vi "CRYConvertWorkinValue.vi"(6 "no ppk?":bool=TRUE, 8 "Work in":u16, 10 "In":T1={"Name"="", "Curve"=[], "X data"=1, "Y data"=1, "Z data"=1, "X axis"=0, "Y axis"=1, "Z axis"=1, "X unit"="Hz", "Y unit"="", "Z unit"="deg.", "X dB ref"=1.0, "Y dB ref"=1.0, "Z dB ref"=1.0, "single val"=FALSE, "protected"=FALSE, "display X"=TRUE, "display Y"=TRUE, "display Z"=TRUE, "Test Info"="", "Step No."=0, "Plot Settings"={"Color"=0, "Interpolation"=0, "Point Style"=0, "Line Style"=0, "Point Color"=0, "Line Width"=0, "Bar Plot Style"=0, "Fill To"=0}, "AutoProtect"=FALSE} {"Z data" items=["dB", "Lin"]; "X data" items=["dB", "Lin"]; "Y data" items=["dB", "Lin"]; "Z dB ref" format="%.1f"; "Z axis" items=["Log", "Lin"]; "X dB ref" format="%.1f"; "X axis" items=["Log", "Lin"]; "Y axis" items=["Log", "Lin"]; "Y dB ref" format="%.1f"; "Curve"."z" format="%.2f"; "Curve"."y" format="%.2f"; "Curve"."x" format="%.2f"}, 11 "Type":u16(slide) caption="Type:") -> (1 "Out":T1={"Name"="", "Curve"=[], "X data"=1, "Y data"=1, "Z data"=1, "X axis"=0, "Y axis"=1, "Z axis"=1, "X unit"="Hz", "Y unit"="", "Z unit"="deg.", "X dB ref"=1.0, "Y dB ref"=1.0, "Z dB ref"=1.0, "single val"=FALSE, "protected"=FALSE, "display X"=TRUE, "display Y"=TRUE, "display Z"=TRUE, "Test Info"="", "Step No."=0, "Plot Settings"={"Color"=0, "Interpolation"=0, "Point Style"=0, "Line Style"=0, "Point Color"=0, "Line Width"=0, "Bar Plot Style"=0, "Fill To"=0}, "AutoProtect"=FALSE} {"Z data" items=["dB", "Lin"]; "X data" items=["dB", "Lin"]; "Y data" items=["dB", "Lin"]; "Z dB ref" format="%.1f"; "Z axis" items=["Log", "Lin"]; "X dB ref" format="%.1f"; "X axis" items=["Log", "Lin"]; "Y axis" items=["Log", "Lin"]; "Y dB ref" format="%.1f"; "Curve"."z" format="%.2f"; "Curve"."y" format="%.2f"; "Curve"."x" format="%.2f"})   [LabVIEW 2013]
uses:
  Typedef Control/CRYData Cluster.ctl
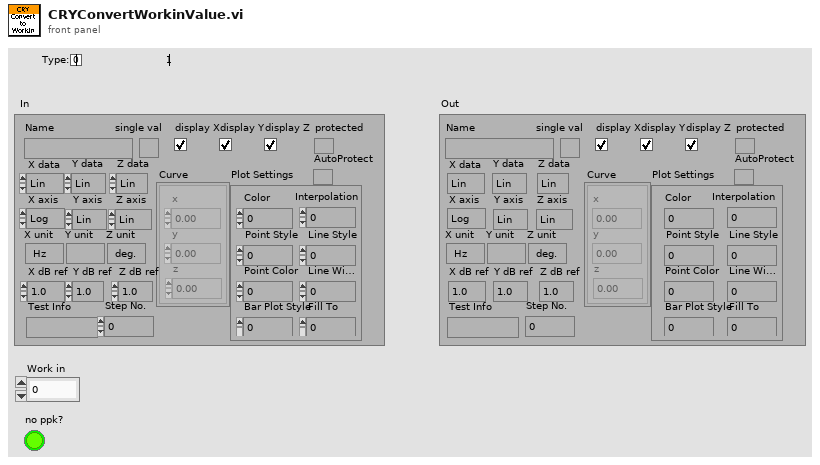
[diagram p1: front panel]
types:
  T1 = typedef "CRYData Cluster.ctl" = cluster{"Name":string, "Curve":cluster{"x":dbl, "y":dbl, "z":dbl}[], "X data":u16, "Y data":u16, "Z data":u16, "X axis":u16, "Y axis":u16, "Z axis":u16, "X unit":string, "Y unit":string, "Z unit":string, "X dB ref":dbl, "Y dB ref":dbl, "Z dB ref":dbl, "single val":bool, "protected":bool, "display X":bool, "display Y":bool, "display Z":bool, "Test Info":string, "Step No.":i32, "Plot Settings":cluster{"Color":u32, "Interpolation":u8, "Point Style":u8, "Line Style":u8, "Point Color":u32, "Line Width":u8, "Bar Plot Style":u8, "Fill To":i16}, "AutoProtect":bool}
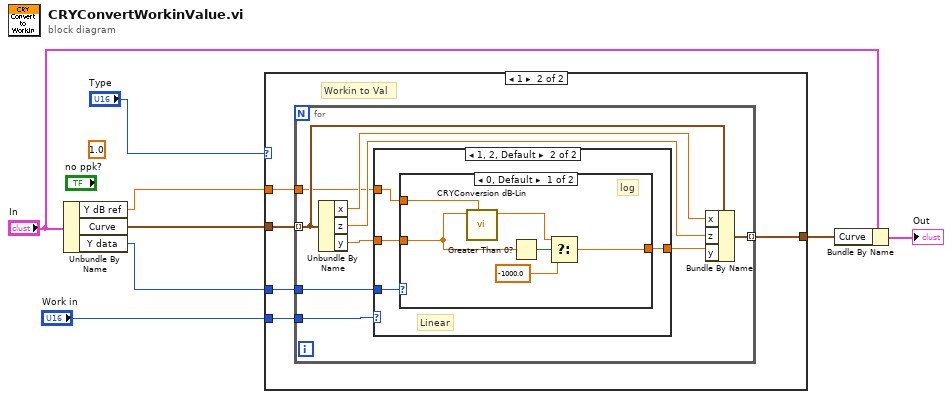
[diagram p0: block diagram]
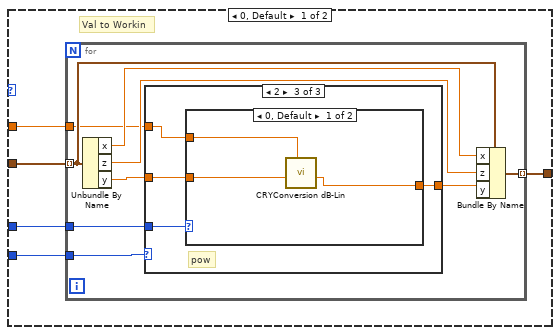
[diagram p2: hidden frame]
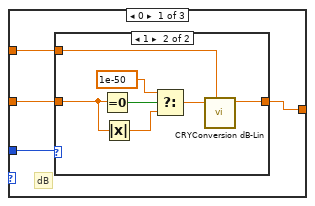
[diagram p3: hidden frame]
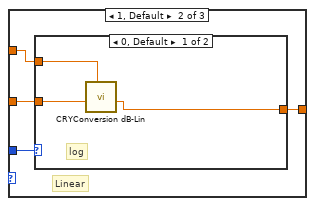
[diagram p5: hidden frame]
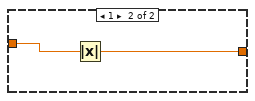
[diagram p7: hidden frame]
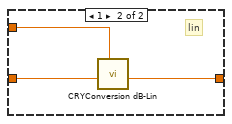
[diagram p9: hidden frame]
diagram:
  (unwired) 1.0 ("Y dB ref")
  n1 = Unbundle By Name("In") -> ("Y dB ref"=w1:dbl, "Curve"=w8:cluster{"x":dbl, "y":dbl, "z":dbl}[], "Y data"=w6:u16)
  n2 = case shown="1" "Type" {
    tunnel: w8 -> [w13 w56]
    tunnel: "Work in" -> [w10 w55]
    tunnel: w6 -> [w11 w54]
    tunnel: [w9 w53] -> w4
    tunnel: w1 -> [w12 w52]
    frame 0, Default {
      # "Val to Workin"
      n3 = for {
        tunnel: w13 -> [w18] mode=indexing
        tunnel: w10 -> [w22]
        tunnel: w11 -> [w20]
        tunnel: [w15] -> w9 mode=indexing
        tunnel: w12 -> [w14]
        n4 = Unbundle By Name(w18) -> ("x"=w19:dbl, "z"=w17:dbl, "y"=w21:dbl)
        n5 = case shown="2" w22 {
          tunnel: w21 -> [w26 w36 w43]
          tunnel: [w25 w37 w45] -> w16
          tunnel: w20 -> [w24 w38 w46]
          tunnel: w14 -> [w23 w35 w44]
          frame 0 {
            # "dB"
            n6 = case shown="1" w24 {
              tunnel: w26 -> [w27 w32]
              tunnel: [w27 w28] -> w25
              tunnel: w23 -> [_ w31]
              frame 0, Default {
              }
              frame 1 {
                n7 = Equal To 0?(x=w32) -> (x = 0?=w34:bool)
                n8 = Absolute Value(x=w32) -> (abs(x)=w30:dbl)
                n9 = Select(t=1e-50, s=w34, f=w30) -> (s? t:f=w29:dbl)
                n10 = call "CRYConversion dB-Lin.vi"("dB ref."=w31, "Lin In"=w29) -> ("Log Out"=w28:dbl)  [unwired: 4 in, 3 out]
              }
            }
          }
          frame 1, Default {
            # "Linear"
            n11 = case shown="0, Default" w38 {
              tunnel: [w39 w42] -> w37
              tunnel: w36 -> [w40 w42]
              tunnel: w35 -> [w41 _]
              frame 0, Default {
                # "log"
                n12 = call "CRYConversion dB-Lin.vi"("dB ref."=w41, "Log In"=w40) -> ("Lin Out"=w39:dbl)  [unwired: 4 in, 3 out]
              }
              frame 1 {
                # "lin"
              }
            }
          }
          frame 2 {
            # "pow"
            n13 = case shown="0, Default" w46 {
              tunnel: [w47 w50] -> w45
              tunnel: w43 -> [w48 w51]
              tunnel: w44 -> [w49 _]
              frame 0, Default {
                n14 = call "CRYConversion dB-Lin.vi"("dB ref."=w49, "Log In"=w48) -> ("Lin Out"=w47:dbl)  [unwired: 4 in, 3 out]
              }
              frame 1 {
                n15 = Absolute Value(x=w51) -> (abs(x)=w50:dbl)
              }
            }
          }
        }
        n16 = Bundle By Name(cluster=w18, "x"=w19, "z"=w17, "y"=w16) -> (w15:cluster{"x":dbl, "y":dbl, "z":dbl})
      }
    }
    frame 1 {
      # "Workin to Val"
      n17 = for {
        tunnel: w56 -> [w61] mode=indexing
        tunnel: w55 -> [w65]
        tunnel: w54 -> [w63]
        tunnel: [w58] -> w53 mode=indexing
        tunnel: w52 -> [w57]
        n18 = Unbundle By Name(w61) -> ("x"=w62:dbl, "z"=w60:dbl, "y"=w64:dbl)
        n19 = case shown="1, 2, Default" w65 {
          tunnel: w64 -> [w69 w75]
          tunnel: [w68 w76] -> w59
          tunnel: w63 -> [w67 w77]
          tunnel: w57 -> [w66 w74]
          frame 0 {
            # "dB"
            n20 = case shown="0, Default" w67 {
              tunnel: w69 -> [w70 w72]
              tunnel: [w70 w71] -> w68
              tunnel: w66 -> [_ w73]
              frame 0, Default {
                # "log"
              }
              frame 1 {
                # "lin"
                n21 = call "CRYConversion dB-Lin.vi"("dB ref."=w73, "Log In"=w72) -> ("Lin Out"=w71:dbl)  [unwired: 4 in, 3 out]
              }
            }
          }
          frame 1, 2, Default {
            # "Linear"
            n22 = case shown="0, Default" w77 {
              tunnel: [w78 w84] -> w76
              tunnel: w75 -> [w81 w84]
              tunnel: w74 -> [w83 _]
              frame 0, Default {
                # "log"
                n23 = call "CRYConversion dB-Lin.vi"("dB ref."=w83, "Lin In"=w81) -> ("Log Out"=w80:dbl)  [unwired: 4 in, 3 out]
                n24 = Greater Than 0?(x=w81) -> (x > 0?=w82:bool)
                n25 = Select(t=w80, s=w82, f=-1000.0) -> (s? t:f=w78:dbl)
              }
              frame 1 {
              }
            }
          }
        }
        n26 = Bundle By Name(cluster=w61, "x"=w62, "z"=w60, "y"=w59) -> (w58:cluster{"x":dbl, "y":dbl, "z":dbl})
      }
    }
  }
  n27 = Bundle By Name(cluster="In", "Curve"=w4) -> (→"Out":T1)
